vi "Query Replay Screen.vi"(8 "error in (no error)":errorcluster, 11 "VISA resource name":refnum<visa-resource-name>) -> (0 "error out":errorcluster, 1 "Screen Index":i32, 2 "Screen Number":i32, 3 "VISA resource name out":refnum<visa-resource-name>)   [LabVIEW 2014, in "Fluke 190 Series II.lvlib"]
doc: "Queries the instrument for the total number of valid replay screens available."
uses:
  Fluke 190 Series II.lvlib
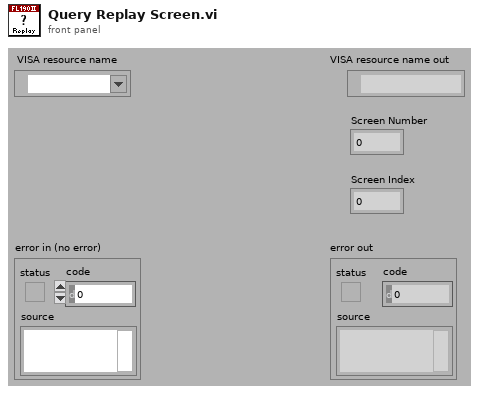
[diagram p1: front panel]
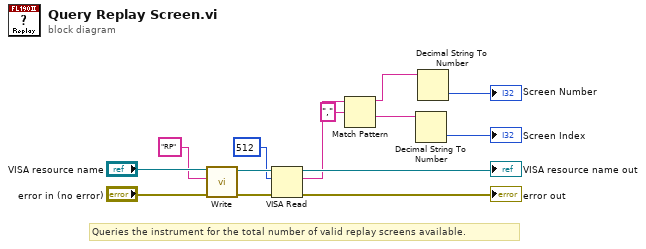
[diagram p0: block diagram]
diagram:
  # "Queries the instrument for the total number of valid replay screens available."
  n1 = call "Write.vi"("error in (no error)"="error in (no error)", "Write Buffer"="RP", "VISA resource name"="VISA resource name") -> ("error out"=w12:errorcluster, "VISA resource name out"=w11:refnum<visa-resource-name>)  [unwired: 7 out]
  n2 = VISA Read(VISA resource name=w11, byte count=u32 512, error in (no error)=w12) -> (VISA resource name out=→"VISA resource name out":refnum<visa-resource-name>, read buffer=w6:string, error out=→"error out":errorcluster)  [unwired: 1 out]
  n3 = Match Pattern(string=w6, regular expression=",") -> (before substring=w4:string, after substring=w2:string)  [unwired: 3 out]
  n4 = Decimal String To Number(string=w2) -> (number=→"Screen Index":i32)  [unwired: 3 out]
  n5 = Decimal String To Number(string=w4) -> (number=→"Screen Number":i32)  [unwired: 3 out]
